vi "Calibrate Current Sense Resistiviy.vi"(0 "DMM ref in":refnum<visa-resource-name>="USB0::0x2A8D::0x0101::MY59004074::INSTR", 2 "Measured Current Sense Resistivity REF":refnum<vi>, 3 "Calibrate Stop REF":refnum<vi>, 5 "DMM error in":errorcluster, 7 "Channel  Count":i32, 8 "Current Sense \nResitance Array\nREF":refnum<vi>, 9 "ESP32 ref in":refnum<visa-resource-name>="COM4", 11 "ESP32 error in":errorcluster, 12 "Manual Trigger Delay (1 s)":dbl=0.0001, 14 "Time out count REF":refnum<vi>) -> (10 "ESP32 ref out":refnum<visa-resource-name>, 15 "ESP32 error out":errorcluster)   [LabVIEW 2023]
uses:
  <instrlib>/Agilent 3446X Series/Agilent 3446X Series.lvlib
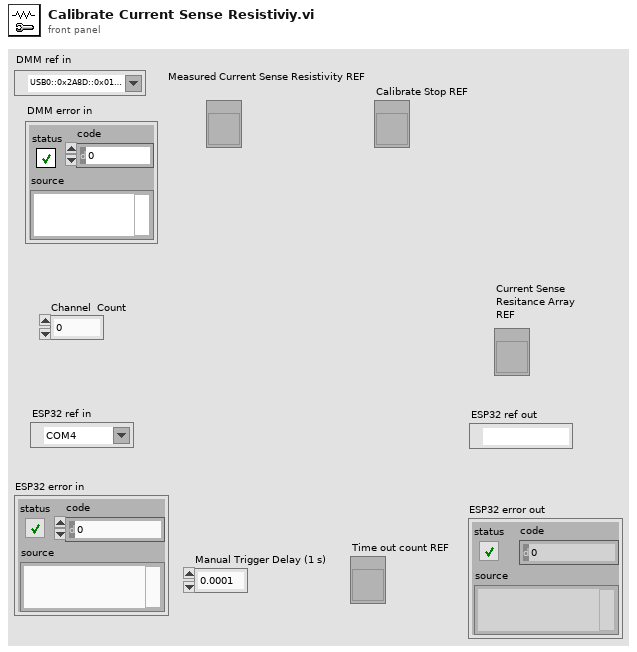
[diagram p1: front panel]
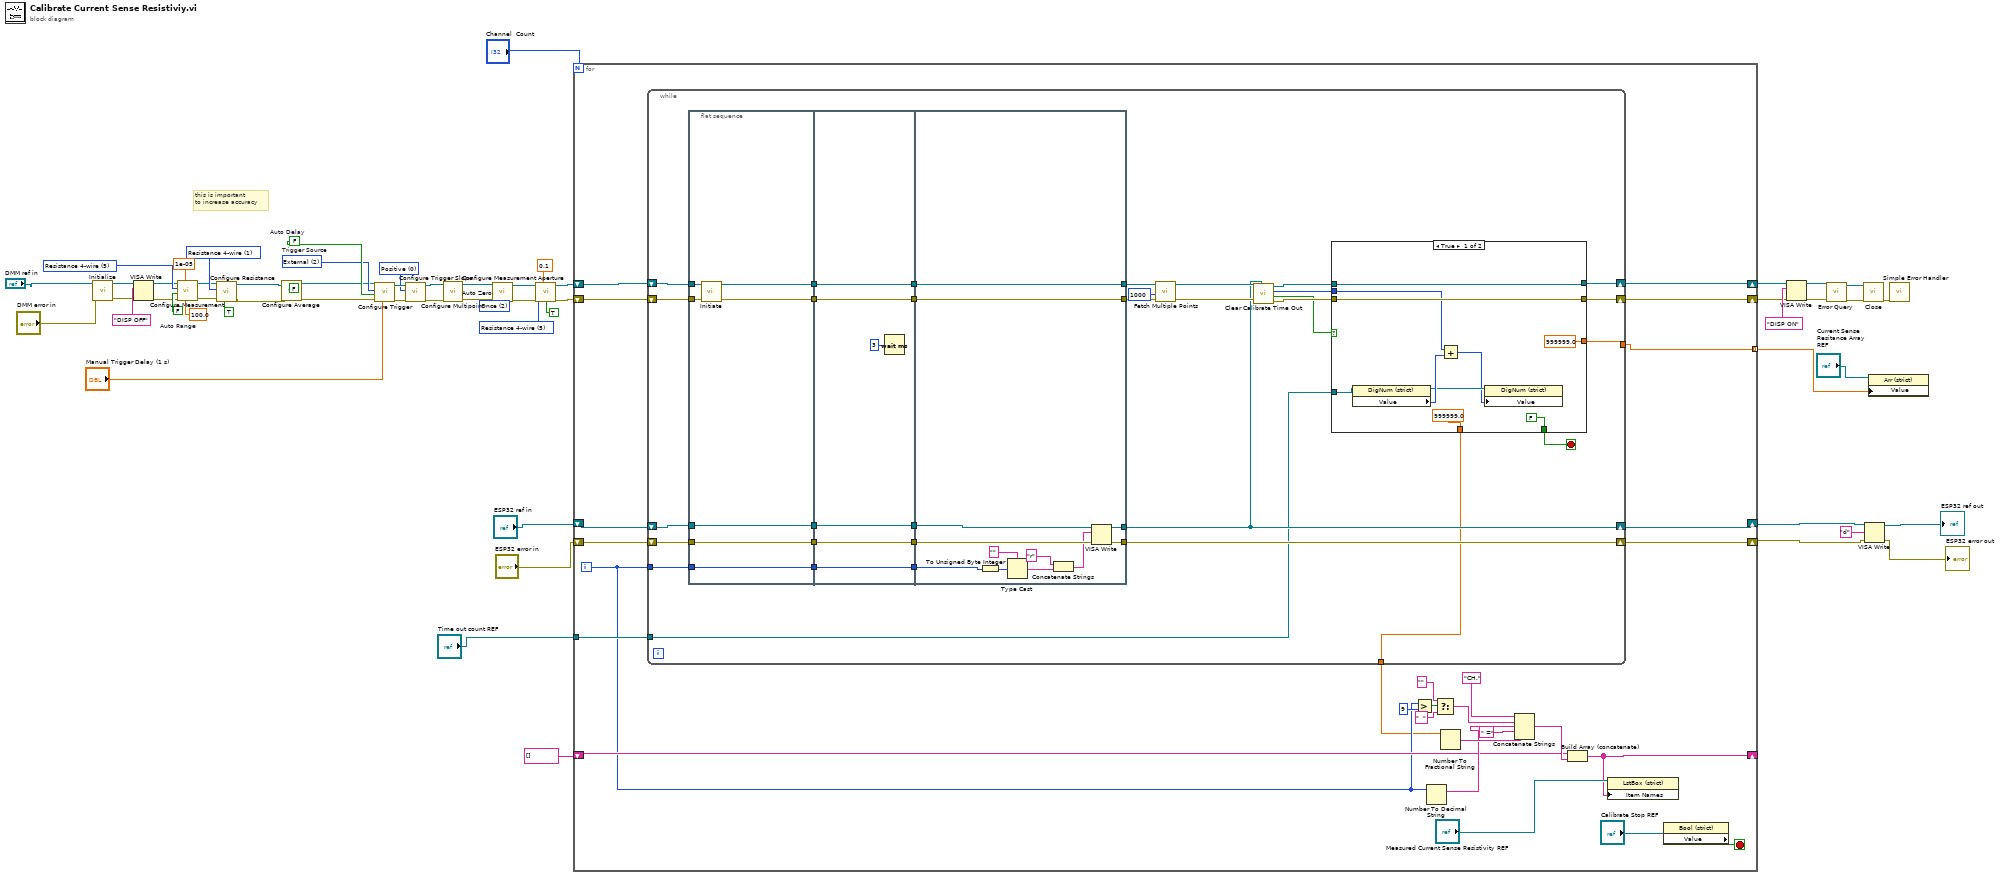
[diagram p0: block diagram]
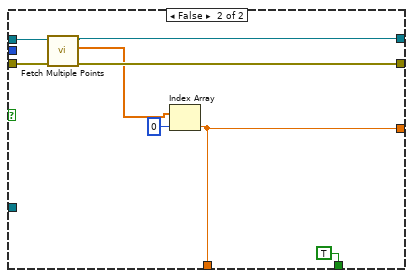
[diagram p2: hidden frame]
diagram:
  w37 = 0 items=["Positive", "Negative"] ("Trigger Edge (1: Negative)")
  w35 = 2 items=["Immediate", "Software (Bus)", "External"]  # Trigger Source
  w36 = FALSE  # Auto Delay
  w45 = 5 items=["Continuity", "Current AC", "Current DC", "Diode", "Frequency", "Resistance 4-wire", "Period", "Resistance 2-wire", "Temperature", "Voltage AC", "Voltage DC", "Voltage DC Ratio", "Capacitance"] ("Measurement Function (10: Voltage DC)")
  w49 = 1 items=["Resistance 2-wire", "Resistance 4-wire"] ("Resistance Type (0: Resistance 2-wire)")
  w51 = 5 items=["Continuity", "Current AC", "Current DC", "Diode", "Frequency", "Resistance 4-wire", "Period", "Resistance 2-wire", "Temperature", "Voltage AC", "Voltage DC", "Voltage DC Ratio", "Capacitance"] ("Measurement Function (0: Continuity)")
  w55 = 2 items=["Disable", "Enable", "Once"] ("Auto Zero (1: Enable)")
  w58 = FALSE  # Auto Range
  # "this is important \nto increase accuracy"
  n1 = call <instrlib>:"Initialize.vi"("error in (no error)"="DMM error in", "VISA resource name"="DMM ref in") -> ("error out"=w21:errorcluster, "VISA resource name out"=w23:refnum<visa-resource-name>)  [unwired: 3 in, 5 out]
  n2 = VISA Write(VISA resource name=w23, write buffer="DISP OFF", error in (no error)=w21) -> (VISA resource name out=w22:refnum<visa-resource-name>, error out=w20:errorcluster)  [unwired: 1 out]
  n3 = call <instrlib>:"Configure Measurement.vi"("Manual Range (1)"=100.0, "Absolute Resolution (1E-6)"=1e-05, "error in (no error)"=w20, "Auto Range (T: Enable)"=w58, "Measurement Function (10: Voltage DC)"=w45, "VISA resource name"=w22) -> ("error out"=w46:errorcluster, "VISA resource name out"=w47:refnum<visa-resource-name>)  [unwired: 4 out]
  n4 = call <instrlib>:"Configure Resistance.vi"("Enable Offset Compensation (F: Disable)"=TRUE, "error in (no error)"=w46, "Resistance Type (0: Resistance 2-wire)"=w49, "VISA resource name"=w47) -> ("error out"=w32:errorcluster, "VISA resource name out"=w33:refnum<visa-resource-name>)  [unwired: 6 in]
  n5 = call <instrlib>:"Configure Average.vi"("error in (no error)"=w32, "Enable Statistics (F: Disable)"=FALSE, "VISA resource name"=w33) -> ("error out"=w30:errorcluster, "VISA resource name out"=w31:refnum<visa-resource-name>)  [unwired: 7 in]
  n6 = call <instrlib>:"Configure Trigger.vi"("Manual Trigger Delay (1 s)"="Manual Trigger Delay (1 s)", "error in (no error)"=w30, "Auto Delay (F:Disable)"=w36, "Trigger Source (0: Immediate)"=w35, "VISA resource name"=w31) -> ("error out"=w39:errorcluster, "VISA resource name out"=w38:refnum<visa-resource-name>)  [unwired: 1 in, 4 out]
  n7 = call <instrlib>:"Configure Trigger Slope.vi"("error in (no error)"=w39, "Trigger Edge (1: Negative)"=w37, "VISA resource name"=w38) -> ("error out"=w28:errorcluster, "VISA resource name out"=w29:refnum<visa-resource-name>)  [unwired: 7 in]
  n8 = call <instrlib>:"Configure Multipoint.vi"("error in (no error)"=w28, "VISA resource name"=w29) -> ("error out"=w26:errorcluster, "VISA resource name out"=w27:refnum<visa-resource-name>)  [unwired: 5 in, 3 out]
  n9 = call <instrlib>:"Auto Zero.vi"("error in (no error)"=w26, "Auto Zero (1: Enable)"=w55, "VISA resource name"=w27) -> ("error out"=w54:errorcluster, "VISA resource name out"=w53:refnum<visa-resource-name>)  [unwired: 7 in]
  n10 = call <instrlib>:"Configure Measurement Aperture.vi"("Aperture Time (0.1s)"=0.1, "error in (no error)"=w54, "Enable Aperture (F: Disable)"=TRUE, "Measurement Function (0: Continuity)"=w51, "VISA resource name"=w53) -> ("error out"=w43:errorcluster, "VISA resource name out"=w44:refnum<visa-resource-name>)  [unwired: 5 in]
  n11 = for {
    N: "Channel  Count" -> [_]
    shift-right: [w83] -> w7
    shift-left: "ESP32 ref in" -> [w85]
    shift-right: [w82] -> w6
    shift-left: "ESP32 error in" -> [w84]
    shift-right: [w78] -> w8
    shift-left: w43 -> [w80]
    shift-right: [w79] -> w9
    shift-left: w44 -> [w81]
    tunnel: "Time out count REF" -> [w77]
    shift-right: [w60] -> _
    shift-left: string[] [] -> [w64]
    tunnel: [w59] -> w2 mode=indexing
    i -> [w63]
    stop <- w75 stop-if-true
    n12 = while {
      tunnel: w63 -> [w104]
      shift-right: [w90] -> w83
      shift-left: w85 -> [w107]
      shift-right: [w105] -> w82
      shift-left: w84 -> [w106]
      shift-right: [w101] -> w79
      shift-left: w81 -> [w103]
      shift-right: [w100] -> w78
      shift-left: w80 -> [w102]
      tunnel: w77 -> [w88]
      tunnel: [w87] -> w62
      tunnel: [w86] -> w59
      stop <- w96 stop-if-true
      n13 = flat-sequence {
        tunnel: w104 -> [w140]
        tunnel: w106 -> [w141]
        tunnel: w107 -> [w142]
        tunnel: [w142] -> w117
        tunnel: [w141] -> w116
        tunnel: [w140] -> w115
        tunnel: w103 -> [w139]
        tunnel: w102 -> [w138]
        tunnel: [w137] -> w114
        tunnel: [w136] -> w113
        tunnel: [w148] -> w112
        tunnel: [w147] -> w111
        tunnel: [w146] -> w110
        tunnel: w117 -> [w148]
        tunnel: w116 -> [w147]
        tunnel: w115 -> [w146]
        tunnel: [w145] -> w109
        tunnel: w114 -> [w145]
        tunnel: [w144] -> w108
        tunnel: w113 -> [w144]
        tunnel: [w158] -> w90
        tunnel: [w154] -> w105
        tunnel: w112 -> [w160]
        tunnel: w111 -> [w159]
        tunnel: w110 -> [w152]
        tunnel: [w151] -> w95
        tunnel: w109 -> [w151]
        tunnel: [w150] -> w94
        tunnel: w108 -> [w150]
        frame #0 {
          n14 = call <instrlib>:"Initiate.vi"("error in (no error)"=w138, "VISA resource name"=w139) -> ("error out"=w136:errorcluster, "VISA resource name out"=w137:refnum<visa-resource-name>)  [unwired: 8 out]
        }
        frame #1 {
          n15 = Wait (ms)(milliseconds to wait=u32 3) -> ()  [unwired: 1 out]
        }
        frame #2 {
          n16 = To Unsigned Byte Integer(number=w152) -> (unsigned 8bit integer=w155:u8)
          n17 = Type Cast(type="" ("string"), x=w155) -> (*(type *) &x=w153:string)
          n18 = Concatenate Strings("r" ("data in"), w153) -> (w149:string)
          n19 = VISA Write(VISA resource name=w160, write buffer=w149, error in (no error)=w159) -> (VISA resource name out=w158:refnum<visa-resource-name>, error out=w154:errorcluster)  [unwired: 1 out]
        }
      }
      n20 = call <instrlib>:"Fetch Multiple Points.vi"("error in (no error)"=w94, "Timeout (10000 ms)"=1000, "VISA resource name"=w95) -> ("error out"=w92:errorcluster, "VISA resource name out"=w93:refnum<visa-resource-name>)  [unwired: 1 in, 6 out]
      n21 = call "Clear Calibrate Time Out.vi"("VISA resource name"=w90, "error in (no error)"=w92, "VISA Refnum in"=w93) -> ("error out"=w98:errorcluster, "error?"=w97:bool, "Time out count"=w89:i32, "VISA Refnum out"=w99:refnum<visa-resource-name>)  [unwired: 5 in]
      n22 = case shown="True" w97 {
        tunnel: [w126 w135] -> w101
        tunnel: [w125 w134] -> w100
        tunnel: w99 -> [w126 w131]
        tunnel: w98 -> [w125 w130]
        tunnel: [FALSE TRUE] -> w96
        tunnel: w89 -> [w124 _]
        tunnel: w88 -> [w123 _]
        tunnel: [999999.0 ("Measurement") w128] -> w87
        tunnel: [999999.0 ("Measurement") w128] -> w86
        frame True {
          n23 = property class="DigNum (strict)"(reference=w123) -> (reference out=w121:refnum<vi>, "Value"=w122:i32)  [unwired: 1 in, 1 out]
          n24 = Add(x=w124, y=w122) -> (x+y=w120:i32)
          n25 = property class="DigNum (strict)"(reference=w121, "Value"=w120) -> ()  [unwired: 1 in, 2 out]
        }
        frame False {
          n26 = call <instrlib>:"Fetch Multiple Points.vi"("error in (no error)"=w130, "VISA resource name"=w131) -> ("error out"=w134:errorcluster, "Measurements"=w133:dbl[], "VISA resource name out"=w135:refnum<visa-resource-name>)  [unwired: 7 in]
          n27 = Index Array(array=w133, index=0) -> (element=w128:dbl)
        }
      }
    }
    n28 = Greater?(x=w63, y=9) -> (0:w69:bool)
    n29 = Number To Decimal String(number=w63) -> (decimal integer string=w73:string)  [unwired: 1 in]
    n30 = Select(t="" ("string"), s=w69, f="  " ("string")) -> (s? t:f=w68:string)
    n31 = Number To Fractional String(number=w62) -> (F-format string=w74:string)  [unwired: 3 in]
    n32 = Concatenate Strings("CH." ("string"), w68, w73, " =" ("string"), w74) -> (w65:string)
    n33 = Build Array (concatenate)(w64, w65) -> (w60:string[])
    n34 = property class="LstBox (strict)"(reference="Measured Current Sense Resistivity REF", "Item Names"=w60) -> ()  [unwired: 1 in, 2 out]
    n35 = property class="Bool (strict)"(reference="Calibrate Stop REF") -> ("Value"=w75:bool)  [unwired: 1 in, 2 out]
  }
  n36 = VISA Write(VISA resource name=w9, write buffer="DISP ON", error in (no error)=w8) -> (VISA resource name out=w18:refnum<visa-resource-name>, error out=w17:errorcluster)  [unwired: 1 out]
  n37 = call <instrlib>:"Error Query.vi"("error in (no error)"=w17, "VISA resource name"=w18) -> ("error out"=w42:errorcluster, "VISA resource name out"=w41:refnum<visa-resource-name>)  [unwired: 8 out]
  n38 = call <instrlib>:"Close.vi"("error in (no error)"=w42, "VISA resource name"=w41) -> ("error out"=w40:errorcluster)  [unwired: 9 out]
  n39 = VISA Write(VISA resource name=w7, write buffer="d" ("data in"), error in (no error)=w6) -> (VISA resource name out=→"ESP32 ref out":refnum<visa-resource-name>, error out=→"ESP32 error out":errorcluster)  [unwired: 1 out]
  n40 = property class="Arr (strict)"(reference="Current Sense \nResitance Array\nREF", "Value"=w2) -> ()  [unwired: 1 in, 2 out]
  n41 = call <vilib>:"Simple Error Handler.vi"("error in (no error)"=w40) -> ()  [unwired: 1 in, 8 out]
